vi "InfoTable to JSON.vi"(8 "error in (no error)":errorcluster, 10 "InfoTable":string[][](array[string])=[["name", "description", "units", "min_value", "max_value"]]) -> (0 "error out":errorcluster, 2 "<JSON>":string="{}")   [LabVIEW 2019, in "Help.lvclass"]
doc: "<b>InfoTable</b> is a table.\n- First row: name, description, units, (min_value, min_value)\n- Remainder: values"
uses:
  Help.lvclass
  d796c62a-3fa9-463e-a79a-0ce26122f36d.vi
  <vilib>/JDP Science/JSONtext/Variant to JSON Text.vi
  <vilib>/JDP Science/JSONtext/LVClass Serializer/JSONtext LVClass Serializer.lvclass
  <vilib>/JDP Science/JSONtext/JSONtext.lvlib
panel:
  in  "InfoTable 2":string[][](array[string])
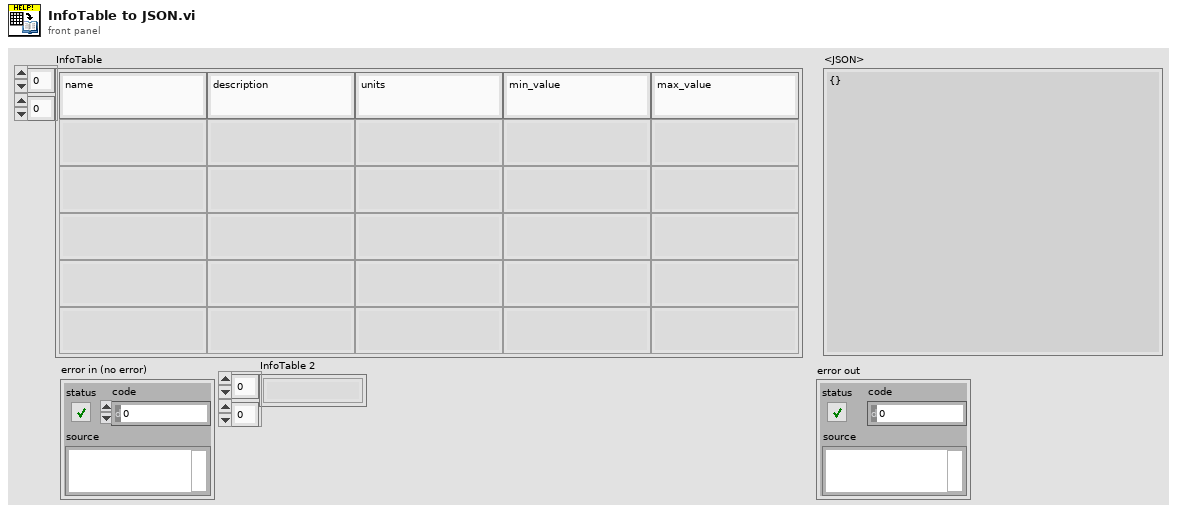
[diagram p1: front panel]
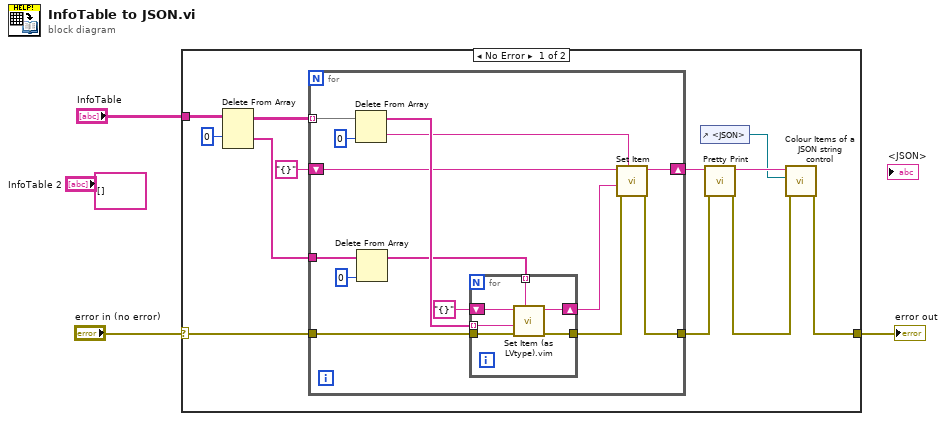
[diagram p0: block diagram]
diagram:
  (unwired) string[][] [] ("InfoTable")
  n1 = case shown="No Error" "error in (no error)" {
    selector: "error in (no error)" -> [w10 w36]
    tunnel: "InfoTable" -> [w15 _]
    tunnel: [w4 w36] -> w1
    frame No Error {
      n2 = Delete From Array(array=w15, index (row)=0) -> (deleted portion=w11:string[], array with subset deleted=w14:string[][])  [unwired: 2 in]
      n3 = for {
        tunnel: w14 -> [w29] mode=indexing
        shift-right: [w23] -> w9
        shift-left: "{}" ("JSON") -> [w24]
        tunnel: w11 -> [w19]
        tunnel: [w21] -> w6
        tunnel: w10 -> [w20]
        n4 = Delete From Array(array=w29, index=0) -> (deleted portion=w25:string, array with subset deleted=w28:string[])  [unwired: 1 in]
        n5 = Delete From Array(array=w19, index=0) -> (array with subset deleted=w18:string[])  [unwired: 1 in, 1 out]
        n6 = for {
          tunnel: w28 -> [w35] mode=indexing
          tunnel: w18 -> [w34] mode=indexing
          shift-right: [w32] -> w27
          shift-left: "{}" ("JSON") -> [w33]
          tunnel: [w31] -> w22
          tunnel: w20 -> [w30]
          n7 = call "Set Item (as LVtype).vim"("$Path or Item Name"=w34, "error in (no error)"=w30, "Anything"=w35, "JSON"=w33) -> ("error out"=w31:errorcluster, "<JSON>"=w32:string)  [unwired: 4 in, 1 out]
        }
        n8 = call <vilib>:"Set Item.vi"("$Path or Item Name"=w25, "error in (no error)"=w22, "JSON to Insert"=w27, "JSON"=w24) -> ("error out"=w21:errorcluster, "<JSON>"=w23:string)  [unwired: 4 in, 1 out]
      }
      n9 = control-ref of="<JSON>"() -> (w7:refnum<vi>)
      n10 = call <vilib>:"Pretty Print.vi"("error in (no error)"=w6, "JSON"=w9) -> ("error out"=w5:errorcluster, "<JSON>"=w8:string)  [unwired: 7 in, 1 out]
      n11 = call <vilib>:"Colour Items of a JSON string control.vi"("error in (no error)"=w5, "String Control"=w7, "JSON"=w8) -> ("error out"=w4:errorcluster)  [unwired: 8 in]
    }
    frame Error {
    }
  }
  "error out" <- w1
